vi "enqueueVisitors.vi"(4 "error in (no error)":errorcluster, 5 "Variable Cluster":T1, 7 "timeout in ms(10)":i32) -> (0 "Event error out":errorcluster, 1 "enqueue failed?":bool[](array[boolean]), 2 "error out":errorcluster, 3 "dup Variable Cluster":T1)   [LabVIEW 2012, in "HGF_SV.lvlib" / "HGF_SVMonitor.lvclass"]
doc: "In case of SV change, this function enqueues the registered network visitors into their target queue along with the new variant data as raw data"
uses:
  HGF_SVMonitor.lvclass
  HGF_BaseClasses/HGF_NetworkVisitor/HGF_NetworkVisitor.lvclass
  HGF_BaseClasses/HGF_TriggeredEvent/HGF_TriggeredEvent.lvclass
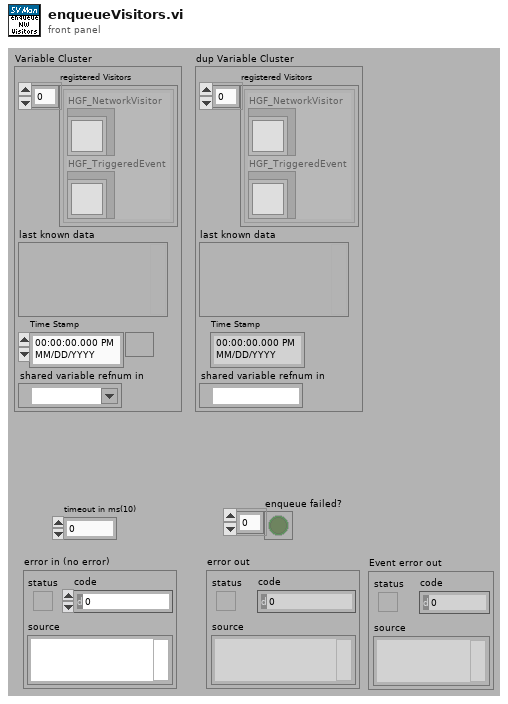
[diagram p1: front panel]
types:
  T1 = cluster{"registered Visitors":cluster{"HGF_NetworkVisitor":refnum<class "HGF_NetworkVisitor.lvclass">, "HGF_TriggeredEvent":refnum<class "HGF_TriggeredEvent.lvclass">}[], "last known data":variant, "Time Stamp":timestamp, "shared variable refnum in":refnum<k21>}
  T2 = cluster{"HGF_NetworkVisitor":refnum<class "HGF_NetworkVisitor.lvclass">, "HGF_TriggeredEvent":refnum<class "HGF_TriggeredEvent.lvclass">}[]
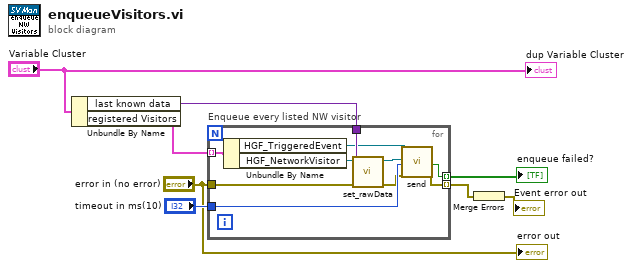
[diagram p0: block diagram]
diagram:
  n1 = Unbundle By Name("Variable Cluster") -> ("last known data"=w7:variant, "registered Visitors"=w8:T2)
  n2 = for "Enqueue every listed NW visitor" {
    tunnel: w8 -> [w18] mode=indexing
    tunnel: w7 -> [w15]
    tunnel: "error in (no error)" -> [w16]
    tunnel: "timeout in ms(10)" -> [w12]
    tunnel: [w9] -> w5 mode=indexing
    tunnel: [w10] -> w4 mode=indexing
    n3 = Unbundle By Name(w18) -> ("HGF_TriggeredEvent"=w14:refnum<class "HGF_TriggeredEvent.lvclass">, "HGF_NetworkVisitor"=w17:refnum<class "HGF_NetworkVisitor.lvclass">)
    n4 = call "set_rawData.vi"("error in (no error)"=w16, "rawData"=w15, "HGF_NetworkData"=w17) -> ("error out"=w11:errorcluster, "dup HGF_NetworkData"=w13:refnum<class "HGF_NetworkVisitor.lvclass">)  [unwired: 7 out]
    n5 = call-dynamic "send.vi"("HGF_Event"=w14, "Object"=w13, "timeout in ms (-1)"=w12, "error in (no error)"=w11) -> ("timed out?"=w10:bool, "error out"=w9:errorcluster)  [unwired: 13 in, 1 out]
  }
  "enqueue failed?" <- w4
  n6 = Merge Errors(w5) -> (→"Event error out":errorcluster)
  "error out" <- "error in (no error)"
  "dup Variable Cluster" <- "Variable Cluster"
